vi "niRFUtil FTW FIR Filter (large real wfm).vi"(0 "Waveform In":T1 {"y" min=0 max=127 format="%.2f"; "dx" format="%^.2e"; "x0" format="%^.2e"}, 5 "Filter":T1 {"y" min=0 max=127 format="%.2f"; "dx" format="%^.2e"; "x0" format="%^.2e"}, 11 "error in (no error)":errorcluster) -> (4 "Waveform Out":T1 {"y" min=0 max=127 format="%.2f"; "dx" format="%^.2e"; "x0" format="%^.2e"}, 15 "error out":errorcluster)   [LabVIEW 2015, in "niRFUtil.lvlib"]
doc: "(c) Copyright 2006, National Instruments, Inc. This VI may not be duplicated, sold, or distributed without written consent from National Instruments."
uses:
  niRFUtil.lvlib
  Includes/niRFUtil INC Real Waveform.ctl
  Includes/niRFUtil INC Real Array.ctl
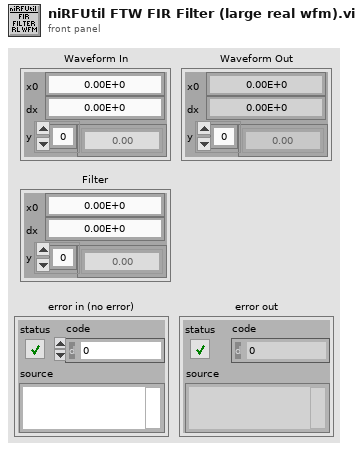
[diagram p1: front panel]
types:
  T1 = typedef "niRFUtil.lvlib/niRFUtil INC Real Waveform.ctl" = cluster{"x0":dbl, "dx":dbl, "y":T2}
  T2 = typedef "niRFUtil.lvlib/niRFUtil INC Real Array.ctl" = sgl[]
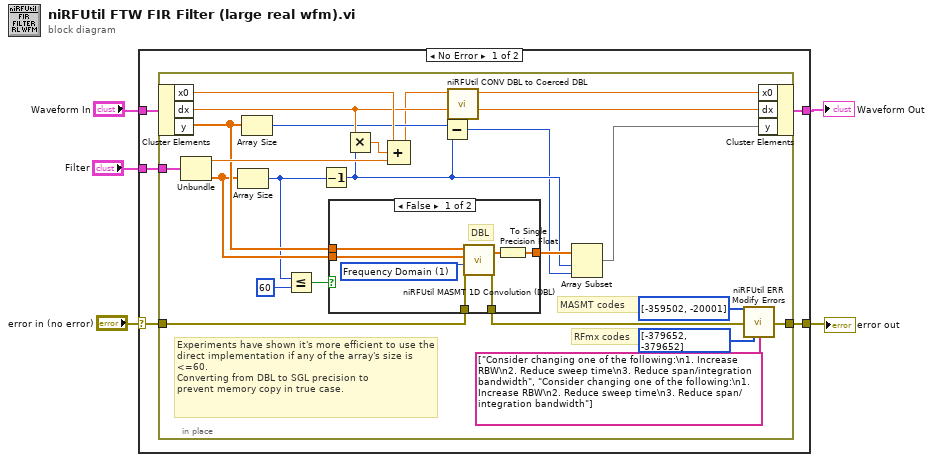
[diagram p0: block diagram]
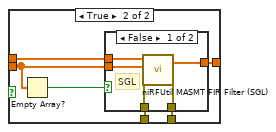
[diagram p2: hidden frame]
diagram:
  n1 = case shown="No Error" "error in (no error)" {
    selector: "error in (no error)" -> [w6 w53]
    tunnel: "Filter" -> [w10 _]
    tunnel: "Waveform In" -> [w9 _]
    tunnel: [w8 _] -> w3
    tunnel: [w7 w53] -> w2
    frame No Error {
      n2 = in-place {
        in-place-border: w10 -> [w31]
        in-place-border: w6 -> [w18]
        in-place-border: [w14] -> w7
        # "RFmx codes"
        # "MASMT codes"
        # "Experiments have shown it's more efficient to use the direct implementation if any of the array's size is <=60. \nConverting from DBL to SGL precision to \nprevent memory copy in true case."
        n3 = in-place-cluster #1(w9) -> ("x0"=w30:dbl, "dx"=w28:dbl, "y"=w29:T2)
        n4 = Unbundle(w31) -> ("x0"=w32:dbl, "y"=w22:T2)  [unwired: 1 out]
        n5 = Array Size(array=w22) -> (size(s)=w19:i32)
        n6 = Array Size(array=w29) -> (size(s)=w24:i32)
        n7 = Less Or Equal?(x=w19, y=60) -> (x <= y?=w21:bool)
        n8 = Decrement(x=w19) -> (x-1=w26:i32)
        n9 = case shown="False" w21 {
          tunnel: [w36 w46] -> w33
          tunnel: w29 -> [w40 w45]
          tunnel: w22 -> [w39 w44]
          tunnel: w18 -> [w35 w41]
          tunnel: [w34 w42] -> w15
          frame False {
            w38 = 1 items=["Direct", "Frequency Domain"] ("algorithm")
            # "DBL"
            n10 = call "niRFUtil MASMT 1D Convolution (DBL).vi"("error in (no error)"=w35, "algorithm"=w38, "Y"=w39, "X"=w40) -> ("error out"=w34:errorcluster, "X * Y"=w37:dbl[])  [unwired: 6 in]
            n11 = To Single Precision Float(number=w37) -> (single precision float=w36:sgl[])
          }
          frame True {
            n12 = Empty Array?(array=w44) -> (empty?=w43:bool)
            n13 = case shown="False" w43 {
              tunnel: [w51 _] -> w46
              tunnel: w45 -> [w50 _]
              tunnel: w44 -> [w49 _]
              tunnel: [w48 w52] -> w42
              tunnel: w41 -> [w47 w52]
              frame False {
                # "SGL"
                n14 = call "niRFUtil MASMT FIR Filter (SGL).vi"("error in (no error)"=w47, "FIR Coefficients"=w49, "X"=w50) -> ("error out"=w48:errorcluster, "Filtered X"=w51:sgl[])  [unwired: 7 in]
              }
              frame True {
              }
            }
          }
        }
        n15 = Multiply(x=w28, y=w26) -> (x*y=w27:dbl)
        n16 = Compound Arithmetic op=ADD(w30, w27, w32) -> (w12:dbl)
        n17 = Subtract(x=w24, y=w26) -> (x-y=w25:i32)
        n18 = call "niRFUtil CONV DBL to Coerced DBL.vi"("Numeric In (DBL)"=w12) -> ("Coerced Numeric Out (DBL)"=w11:dbl)  [unwired: 10 in]
        n19 = Array Subset(array=w33, index=w26, length=w25) -> (w23:sgl[])
        n20 = call "niRFUtil ERR Modify Errors.vi"("Error codes"=i32[] [-359502, -20001], "error in (no error)"=w15, "Modified Error\\Warning Codes"=i32[] [-379652, -379652] ("Modified Error\\Warning Codes"), "Modified Error Source"=string[] ["Consider changing one of the following:\n1. Increase RBW\n2. Reduce sweep time\n3. Reduce span/integration bandwidth", "Consider changing one of the following:\n1. Increase RBW\n2. Reduce sweep time\n3. Reduce span/integration bandwidth"]) -> ("error out"=w14:errorcluster)  [unwired: 11 in]
        n21 = in-place-cluster #1("x0"=w11, "dx"=w28, "y"=w23) -> (w8:T1)
      }
    }
    frame Error {
    }
  }
  "Waveform Out" <- w3
  "error out" <- w2
